vi "Error Module.vi"(7 "Command (Handle Errors":T4=enum."Handle Errors", 8 "error in":errorcluster, 9 "dynamic event queue reference":T3, 10 "User Interface Queue Reference":T2, 11 "User Event Queue Refence":T1) -> (0 "error out":errorcluster, 2 "status":bool)   [LabVIEW 2011]
doc: "Controls access to the Cue data."
uses:
  Error Module Action.ctl
  Controls/Dynamic Event Queue Reference.ctl
  Controls/User Interface Queue Reference.ctl
  Controls/User Interface Control.ctl
  Controls/User Interface Action.ctl
  Controls/User Event Queue Reference.ctl
  Controls/User Event Control.ctl
  Controls/User Event Action.ctl
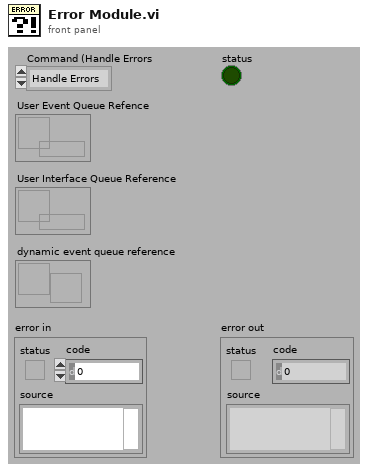
[diagram p1: front panel]
types:
  T1 = typedef "User Event Queue Reference.ctl" = refnum<queue>
  T2 = typedef "User Interface Queue Reference.ctl" = refnum<queue>
  T3 = typedef "Dynamic Event Queue Reference.ctl" = refnum<user-event>
  T4 = typedef "Error Module Action.ctl" = enum16{"Initialize", "Handle Errors", "Report Errors"}
  T5 = typedef "User Interface Control.ctl" = cluster{"action":T6, "data1":variant, "data2":variant}
  T6 = typedef "User Interface Action.ctl" = enum16{"Initialize", "Visibility Front Panel Controls", "Stop"}
  T7 = typedef "User Event Control.ctl" = cluster{"action":T8, "data":variant}
  T8 = typedef "User Event Action.ctl" = enum16{"Initialize", "Device Connections", "Device Settings", "Shutdown"}
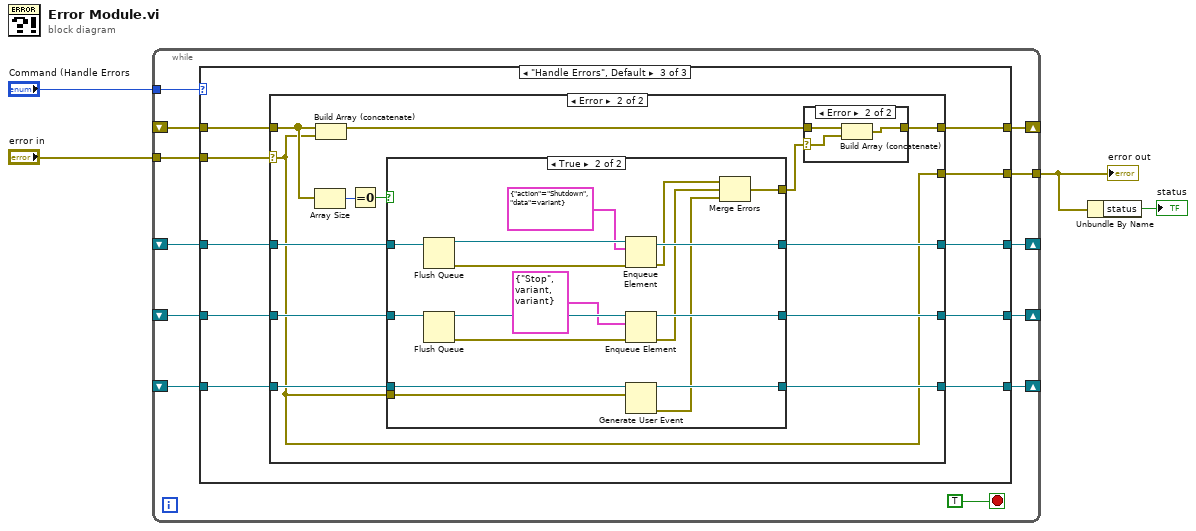
[diagram p0: block diagram]
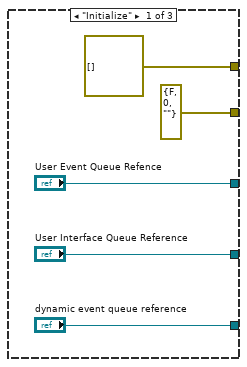
[diagram p2: hidden frame]
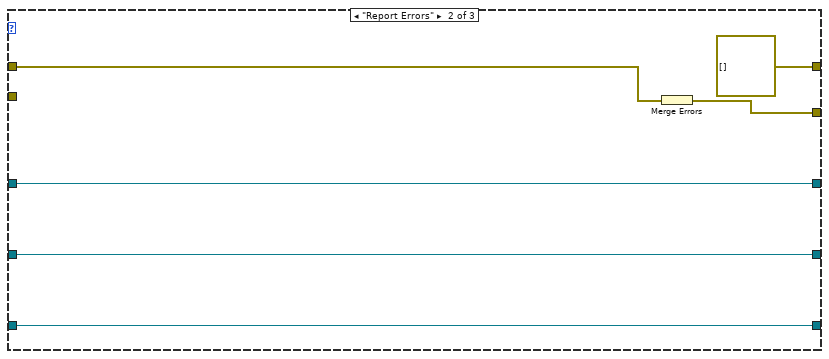
[diagram p3: hidden frame]
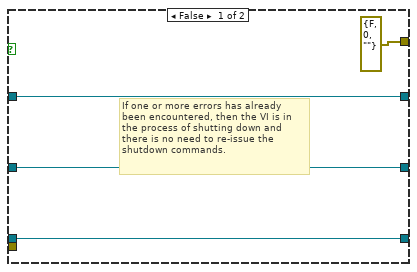
[diagram p6: hidden frame]
diagram:
  n1 = while {
    shift-right: [w12] -> _
    shift-left: _ -> [w14]
    tunnel: "error in" -> [w15]
    tunnel: "Command (Handle Errors" -> [w13]
    tunnel: [w11] -> w2
    shift-right: [w5] -> _
    shift-left: _ -> [w10]
    shift-right: [w6] -> _
    shift-left: _ -> [w9]
    shift-right: [w7] -> _
    shift-left: _ -> [w8]
    stop <- TRUE stop-if-true
    n2 = case shown="\"Handle Errors\", Default" w13 {
      tunnel: w15 -> [_ _ w37]
      tunnel: [errorcluster[] [] errorcluster[] [] w35] -> w12
      tunnel: w14 -> [_ w26 w36]
      tunnel: [errorcluster {"status"=FALSE, "code"=0, "source"=""} ("error out") w27 w28] -> w11
      tunnel: w10 -> [_ w25 w34]
      tunnel: w9 -> [_ w24 w33]
      tunnel: w8 -> [_ w23 w32]
      tunnel: ["dynamic event queue reference" w23 w29] -> w7
      tunnel: ["User Interface Queue Reference" w24 w30] -> w6
      tunnel: ["User Event Queue Refence" w25 w31] -> w5
      frame "Initialize" {
      }
      frame "Report Errors" {
        n3 = Merge Errors(w26) -> (w27:errorcluster)
      }
      frame "Handle Errors", Default {
        n4 = case shown="Error" w37 {
          selector: w37 -> [w38 w43]
          tunnel: [w42 w51] -> w35
          tunnel: w36 -> [w42 w55]
          tunnel: w34 -> [w41 w49]
          tunnel: w33 -> [w40 w48]
          tunnel: w32 -> [w39 w47]
          tunnel: [w39 w46] -> w29
          tunnel: [w40 w45] -> w30
          tunnel: [w41 w44] -> w31
          tunnel: [w38 w43] -> w28
          frame No Error {
          }
          frame Error {
            n5 = Array Size(array=w55) -> (size(s)=w53:i32)
            n6 = Build Array (concatenate)(w55, w43) -> (w52:errorcluster[])
            n7 = Equal To 0?(x=w53) -> (x = 0?=w54:bool)
            n8 = case shown="True" w54 {
              tunnel: [errorcluster {"status"=FALSE, "code"=0, "source"=""} ("error out") w69] -> w50
              tunnel: w43 -> [_ w73]
              tunnel: w49 -> [w62 w80]
              tunnel: w48 -> [w61 w79]
              tunnel: w47 -> [w60 w74]
              tunnel: [w60 w72] -> w46
              tunnel: [w61 w71] -> w45
              tunnel: [w62 w70] -> w44
              frame False {
                # "If one or more errors has already \nbeen encountered, then the VI is in \nthe process of shutting down and \nthere is no need to re-issue the \nshutdown commands."
              }
              frame True {
                n9 = Flush Queue(queue=w80) -> (queue out=w78:T1, error out=w75:errorcluster)  [unwired: 1 in, 1 out]
                n10 = Flush Queue(queue=w79) -> (queue out=w77:T2, error out=w76:errorcluster)  [unwired: 1 in, 1 out]
                n11 = Enqueue Element(queue=w78, element=T7 {"action"=enum."Shutdown", "data"=variant} ("User Event Control"), error in (no error)=w75) -> (queue out=w70:T1, error out=w68:errorcluster)  [unwired: 1 in, 1 out]
                n12 = Enqueue Element(queue=w77, element=T5 {"action"=enum."Stop", "data1"=variant, "data2"=variant} ("User Interface Control"), error in (no error)=w76) -> (queue out=w71:T2, error out=w67:errorcluster)  [unwired: 1 in, 1 out]
                n13 = Generate User Event(user event=w74, event data cluster=w73) -> (user event out=w72:T3, error out=w66:errorcluster)  [unwired: 1 in]
                n14 = Merge Errors(w68, w67, w66) -> (w69:errorcluster)
              }
            }
            n15 = case shown="Error" w50 {
              selector: w50 -> [_ w57]
              tunnel: w52 -> [w56 w59]
              tunnel: [w56 w58] -> w51
              frame No Error {
              }
              frame Error {
                n16 = Build Array (concatenate)(w59, w57) -> (w58:errorcluster[])
              }
            }
          }
        }
      }
    }
  }
  "error out" <- w2
  n17 = Unbundle By Name(w2) -> ("status"=→"status":bool)
